vi "Avoid NaN.vi"(1 "Value":dbl) -> (0 "Number":dbl)   [LabVIEW 2013]
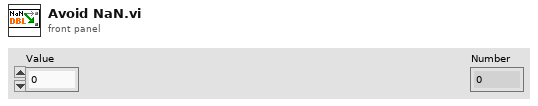
[diagram p1: front panel]
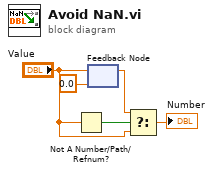
[diagram p0: block diagram]
diagram:
  n1 = Not A Number/Path/Refnum?(number/path/refnum="Value") -> (NaN/Path/Refnum?=w5:bool)
  n2 = feedback #1(0.0 ("Number")) -> (w4:dbl)
  n3 = feedback-in #1("Value") -> ()
  n4 = Select(t=w4, s=w5, f="Value") -> (s? t:f=→"Number":dbl)
